vi "lvsocket read.vi"(8 "error in":errorcluster, 9 "max read size":u64=10000, 11 "tls context":u64) -> (0 "error out":errorcluster, 2 "buffer":string, 3 "error response":i32)   [LabVIEW 2016, in "lv tls dll.lvlib"]
uses:
  lv tls dll.lvlib
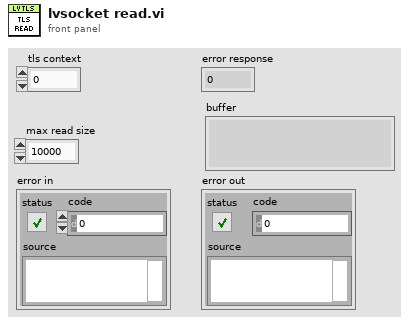
[diagram p1: front panel]
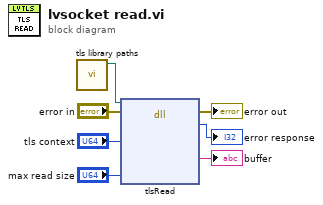
[diagram p0: block diagram]
diagram:
  n1 = call "tls library paths.vi"() -> ("lvtls"=w1:path)  [unwired: 8 in, 3 out]
  n2 = dll-call lib="C:/Users/IEUser/Desktop/tlssimple/lvlibtls.dll" fn="tlsRead"(path in=w1, error in="error in", "context"="tls context", "maxlen"="max read size") -> (error out=→"error out":errorcluster, "return"=→"error response":i32, "data"=→"buffer":string)  [unwired: 4 in, 1 out]
